vi "VI_Heat_Tape_Final_double.vi"() -> ()   [LabVIEW 2019]
uses:
  <vilib>/NI/Modbus Library/API/Wrapper/Create Serial Master.vi
  <vilib>/NI/Modbus Library/API/Master/Modbus Master.lvclass
  <vilib>/NI/Modbus Library/API/Wrapper/API Main.lvlib
  <vilib>/NI/Modbus Library/Transmission Data Unit/RTU/RTU Data Unit.lvclass
panel:
  in  "?":bool
  in  "unit ID (Defaut: 1) 2":u8=1
  in  "error check 2":errorcluster
  in  "Flow Control (Default: None) 2":u16(ring) items=["None", "XON/XOFF", "RTS/CTS", "XON/XOFF & RTS/CTS", "DTR/DSR", "XON/XOFF & DTR/DSR"]
  in  "Serial Type (Default: RTU) 2":enum16{"RTU", "ASCII"}(ring)
  in  "Parity (Default: None) 2":u16(ring)=2 items=["None", "Odd", "Even", "Mark", "Space"]
  in  "Baud Rate (Default: 115400) 2":u32=9600
  in  "COM Port (Default: COM7) 2":refnum<visa-resource-name>
  in  "starting address (Default: 1) 2":u16
  in  "number of inputs (Defaut: 60) 2":u16
  out "Register and RAW value 2":u16[](array[numeric])
  out "Query Message 2":string
  out "Heat Tape 01  Temperature (ºF) 2":dbl(slide) scale=65.0..85.0
  in  "?":bool
  out "Current Temperature (ºF) 2":string
  out "?":cluster{dbl, dbl}(graph)
  in  "Hysterisis Value 2":string
  out "Current Temperature Status 2":bool
  out "Alarm Status 2":bool
  out "Connection Status 2":bool
  in  "Manual/Auto 2":string(combo)
  in  "Set Value 2":string
  in  "Key Lock 2":string(combo)
  in  "Preset 2":string(combo)
  out "Heater Status 2":bool
  in  "Auto Tunning 2":string(combo)
  in  "Control Mode 2":string(combo)
  in  "?":bool
  in  "Normal/Reverse Setting 2":string(combo)
  in  "?":bool
  out "Value 5":sgl
  out "Value 4":sgl
  out "Value 3":sgl
  out "Value 2":sgl
  in  "Normal/Reverse Setting":string(combo)
  in  "Control Mode":string(combo)
  in  "Auto Tunning":string(combo)
  in  "?":bool
  in  "?":bool
  in  "Manual/Auto":string(combo)
  in  "Key Lock":string(combo)
  in  "Set Value":string
  in  "Preset":string(combo)
  in  "Hysterisis Value":string
  out "Connection Status":bool
  in  "unit ID (Defaut: 1)":u8=1
  in  "number of inputs (Defaut: 60)":u16
  in  "starting address (Default: 1)":u16
  in  "Flow Control (Default: None)":u16(ring) items=["None", "XON/XOFF", "RTS/CTS", "XON/XOFF & RTS/CTS", "DTR/DSR", "XON/XOFF & DTR/DSR"]
  in  "Serial Type (Default: RTU)":enum16{"RTU", "ASCII"}(ring)
  in  "Parity (Default: None)":u16(ring)=2 items=["None", "Odd", "Even", "Mark", "Space"]
  in  "Baud Rate (Default: 115400)":u32=9600
  in  "COM Port (Default: COM7)":refnum<visa-resource-name>
  out "Alarm Status":bool
  out "?":cluster{dbl, dbl}(graph)
  out "Heater Status":bool
  out "Current Temperature Status":bool
  in  "?":bool
  out "Current Temperature (ºF)":string
  out "Heat Tape 01  Temperature (ºF)":dbl(slide) scale=65.0..85.0
  out "Query Message":string
  out "Register and RAW value":u16[](array[numeric])
  in  "error check":errorcluster
  # "SpinQuest Heat Tape Temperature Monitoring System"
  # "PXF4 Settings"
  # "RS-485 Connection"
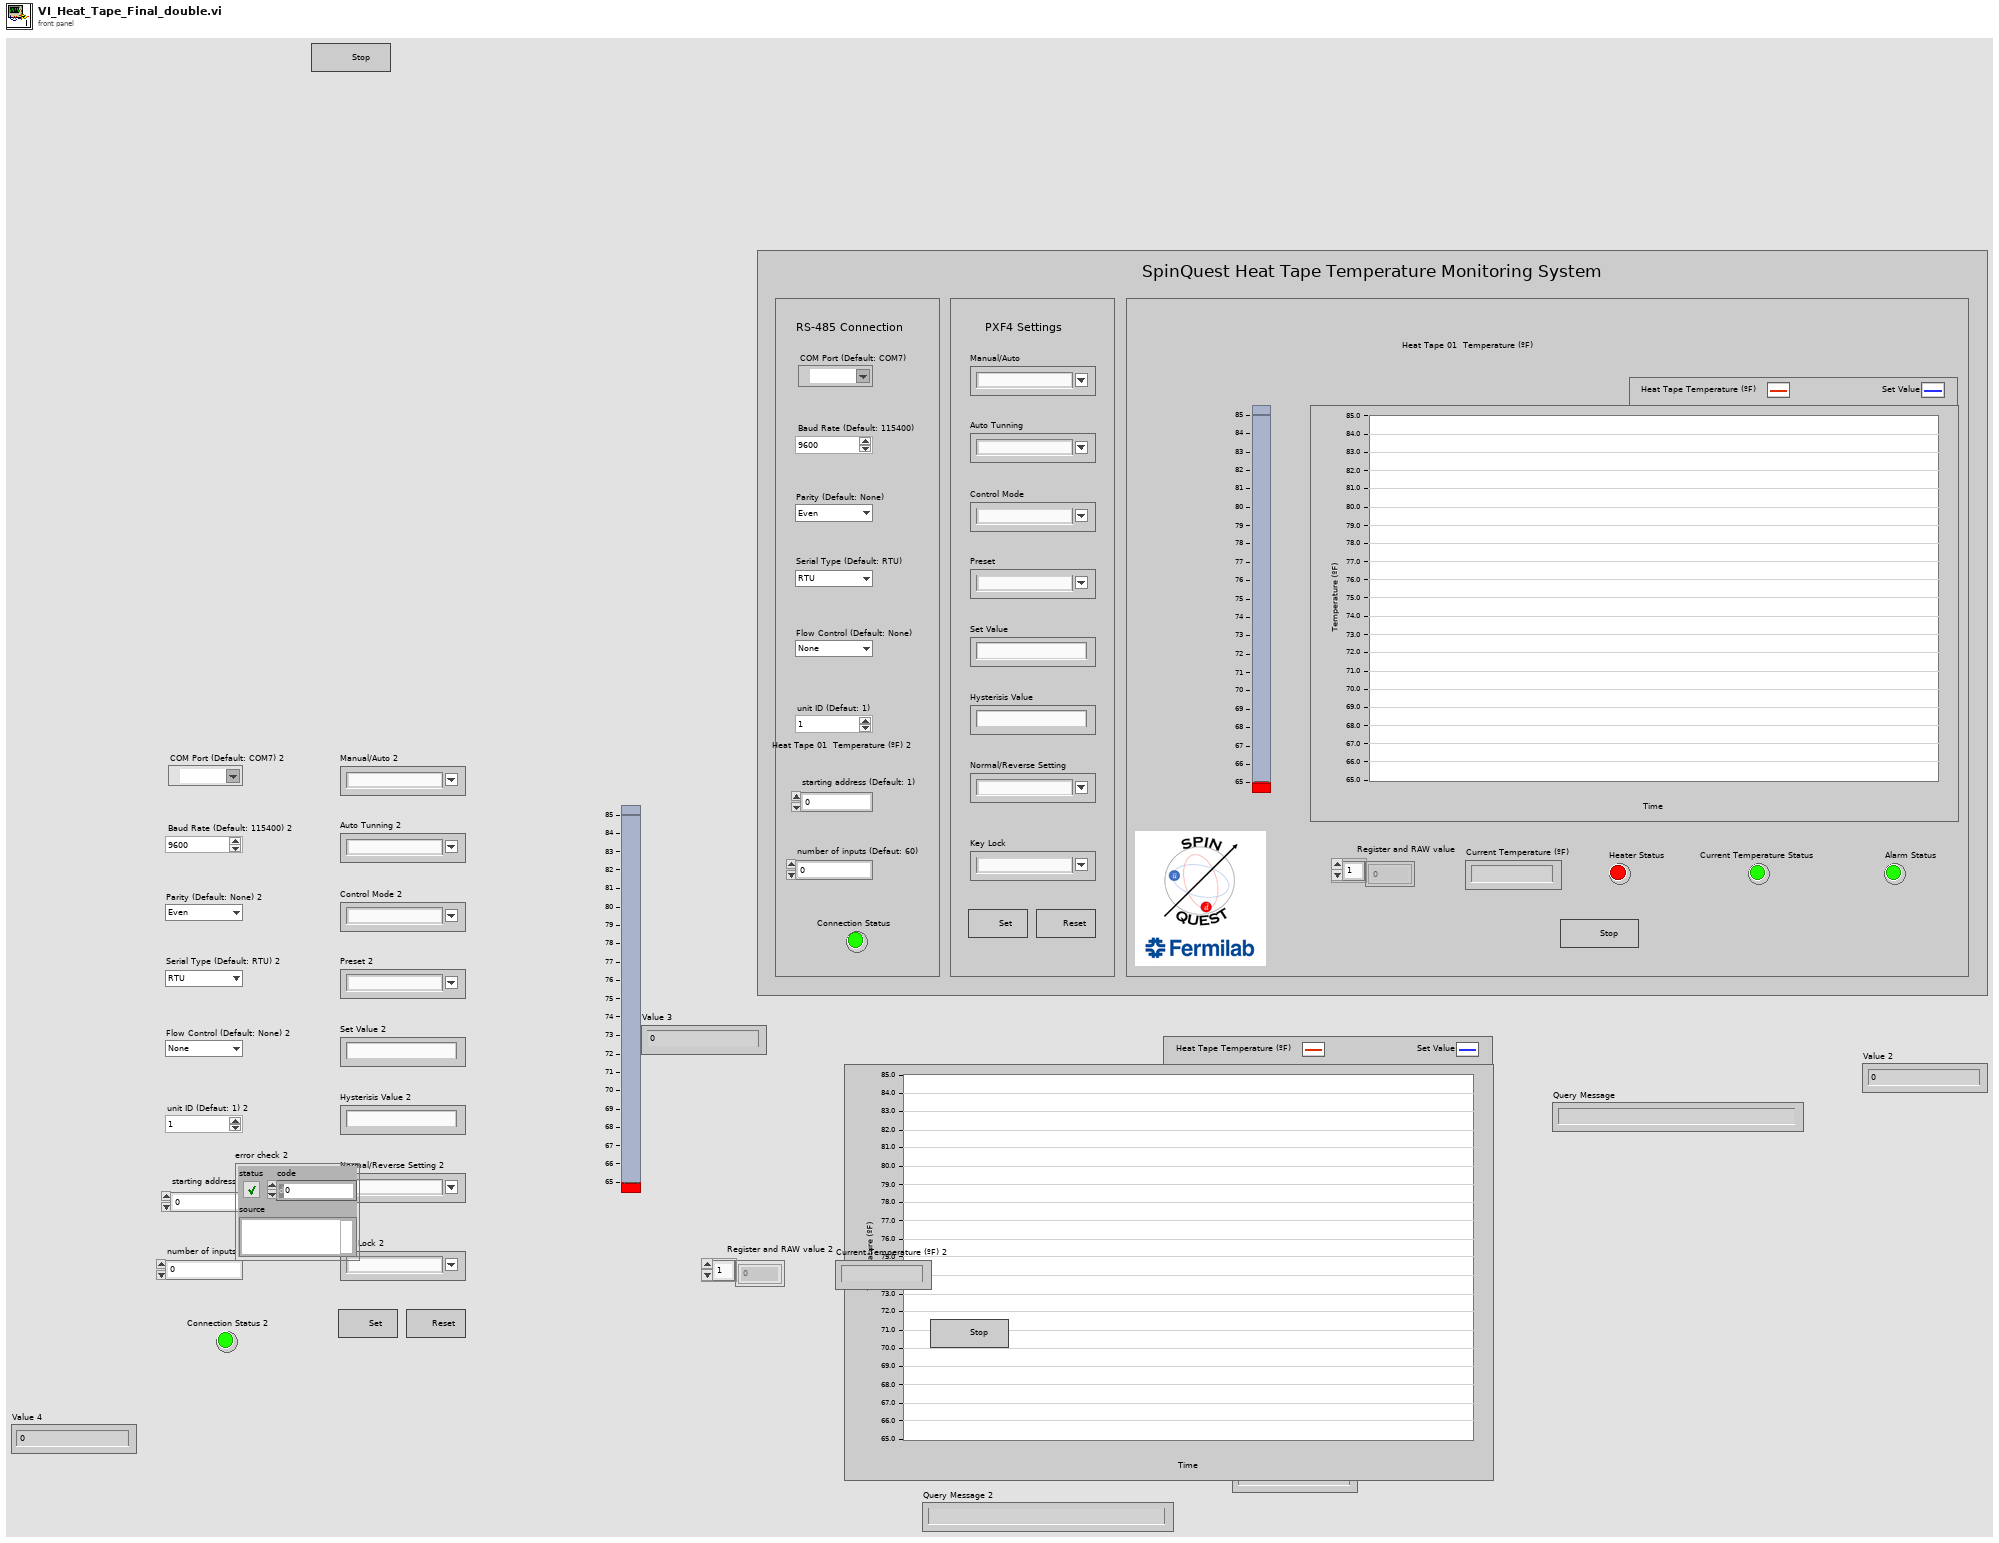
[diagram p1: front panel]
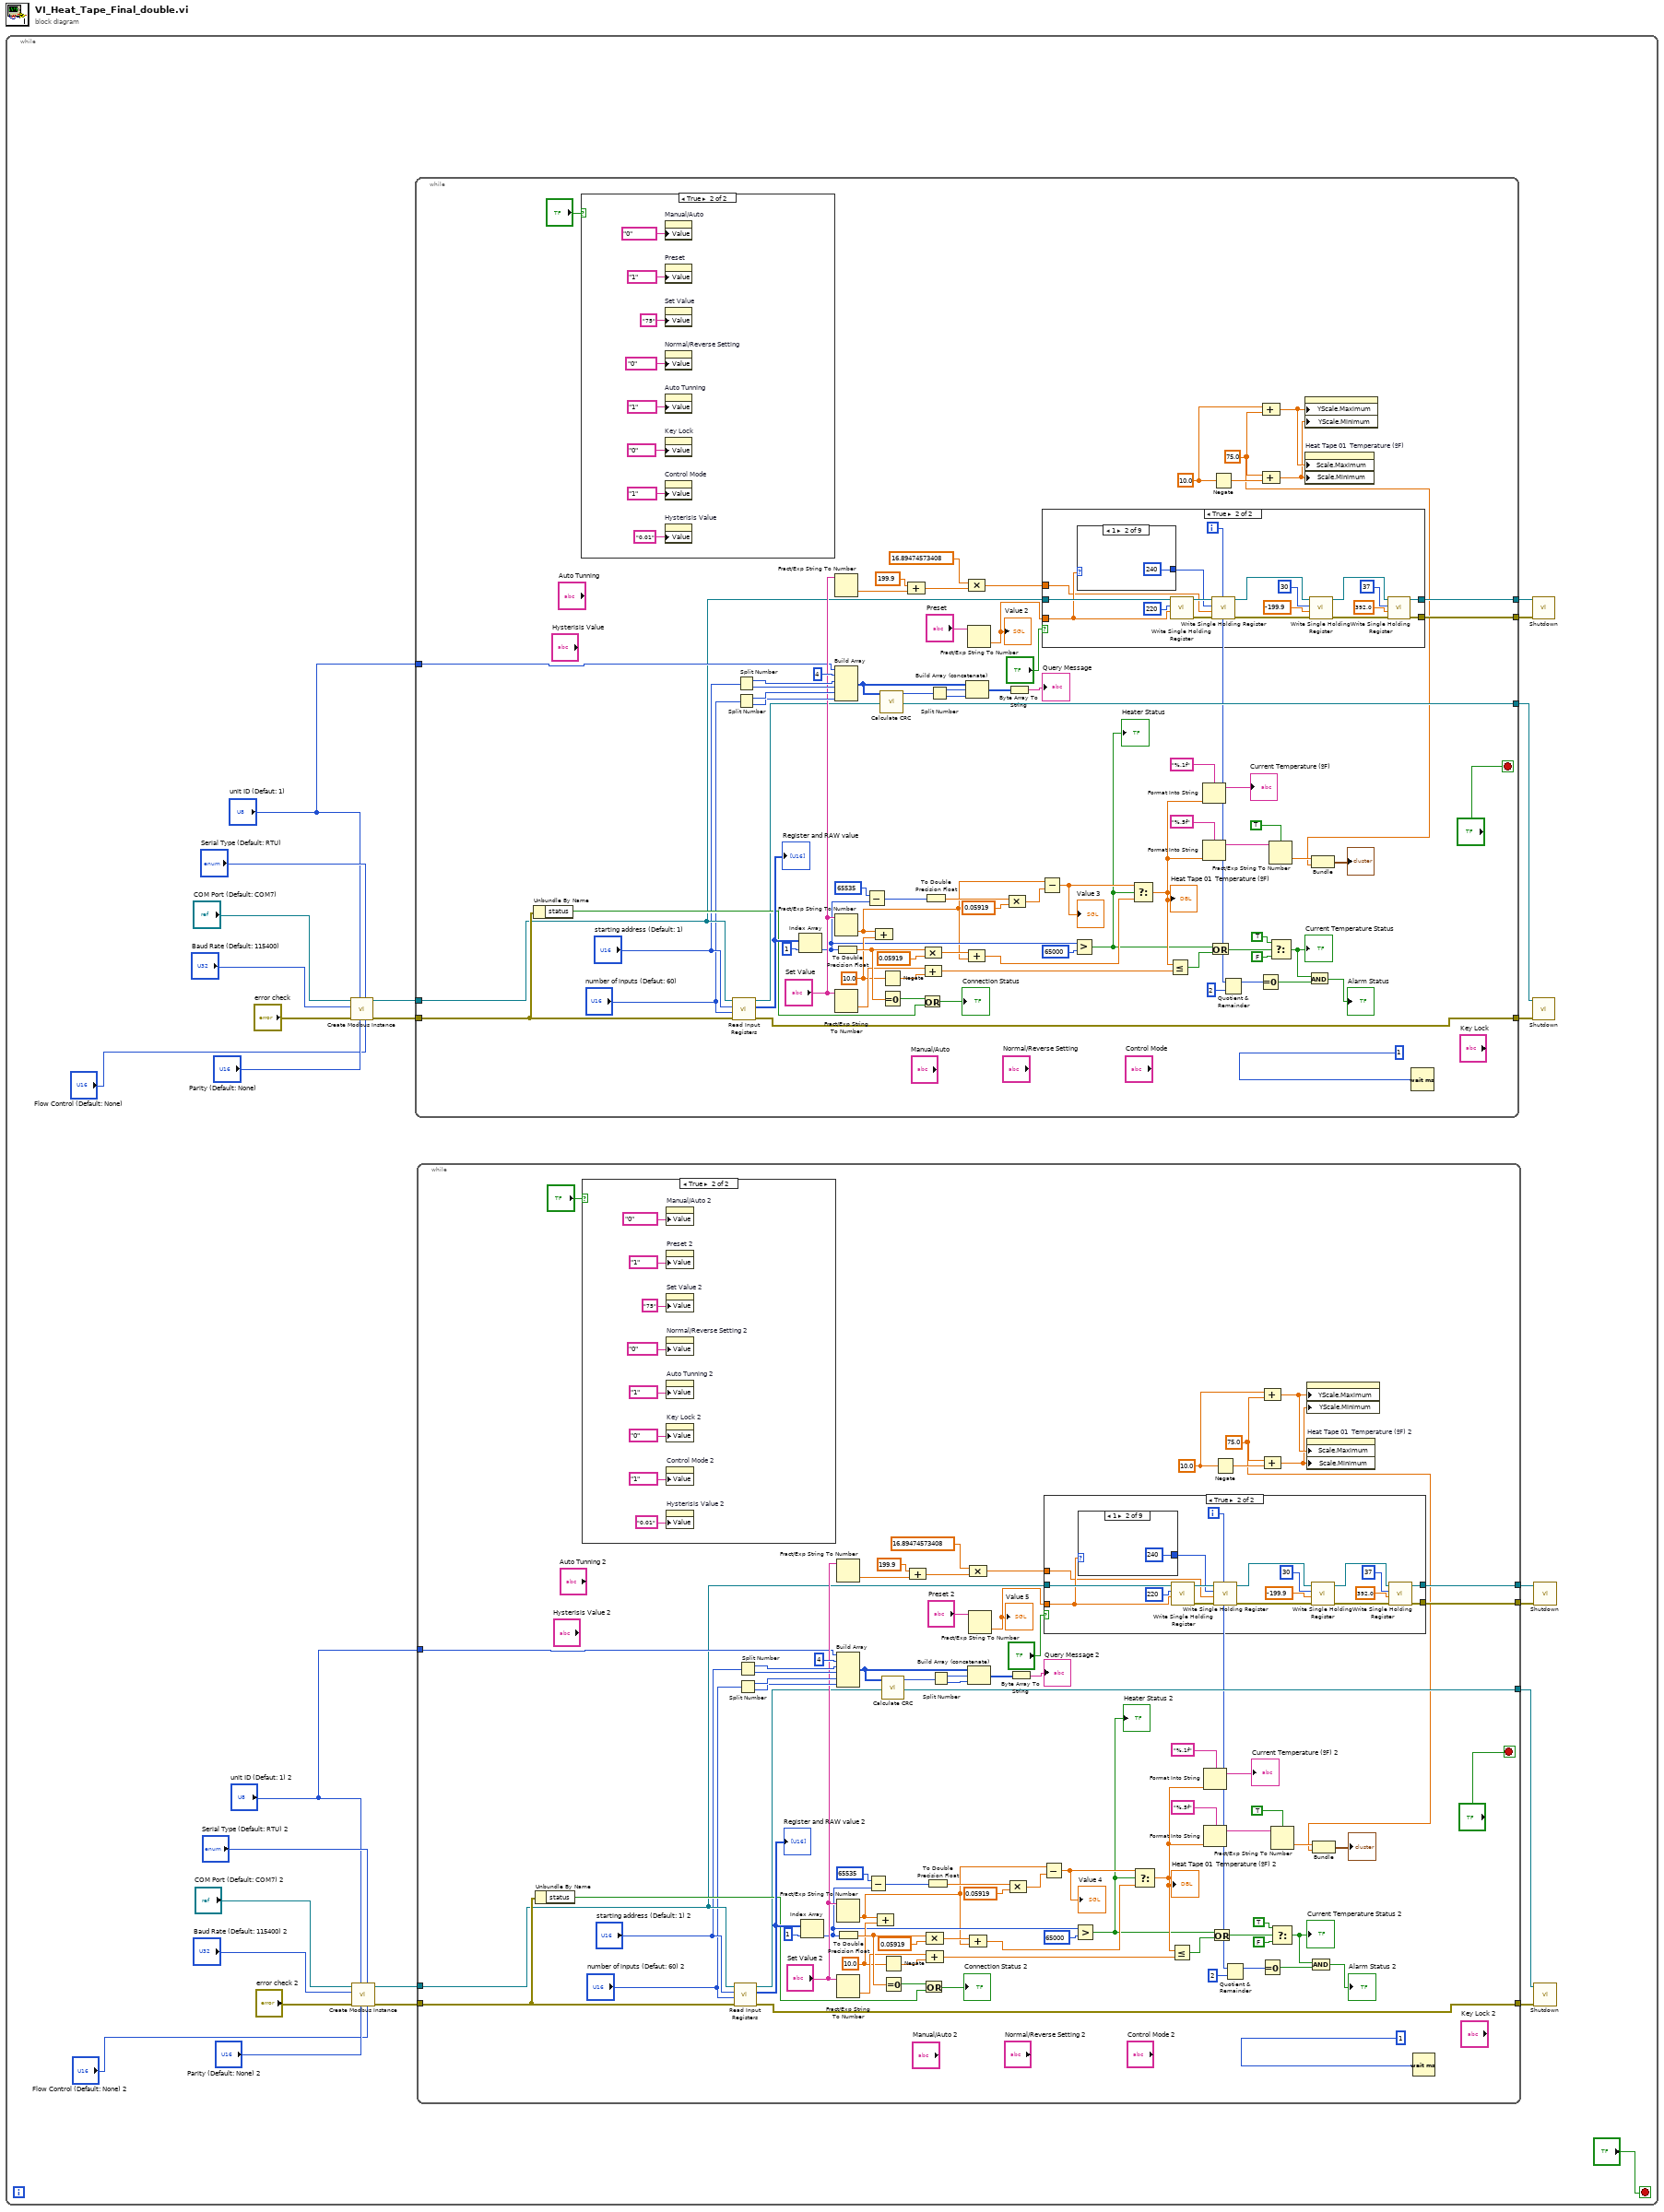
[diagram p0: block diagram]
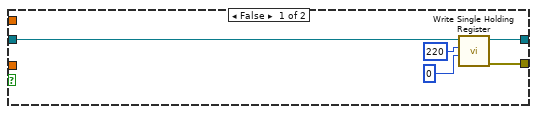
[diagram p2: hidden frame]
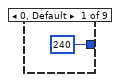
[diagram p3: hidden frame]
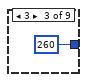
[diagram p4: hidden frame]
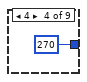
[diagram p5: hidden frame]
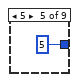
[diagram p6: hidden frame]
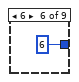
[diagram p7: hidden frame]
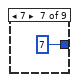
[diagram p8: hidden frame]
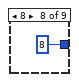
[diagram p9: hidden frame]
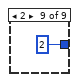
[diagram p10: hidden frame]
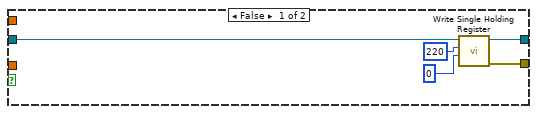
[diagram p12: hidden frame]
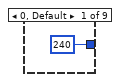
[diagram p13: hidden frame]
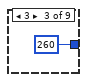
[diagram p14: hidden frame]
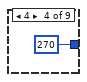
[diagram p15: hidden frame]
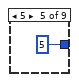
[diagram p16: hidden frame]
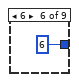
[diagram p17: hidden frame]
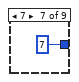
[diagram p18: hidden frame]
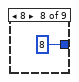
[diagram p19: hidden frame]
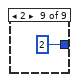
[diagram p20: hidden frame]
diagram:
  n1 = while {
    stop <- "?" stop-if-true
    n2 = call-poly <vilib>:"Create Modbus Instance.vi"("flow control (none)"="Flow Control (Default: None)", "serial type"="Serial Type (Default: RTU)", "parity (even)"="Parity (Default: None)", "unit ID"="unit ID (Defaut: 1)", "error in"="error check", "baud rate"="Baud Rate (Default: 115400)", "VISA resource name"="COM Port (Default: COM7)") -> ("error out"=w21:errorcluster, "serial master instance"=w22:refnum<class "Modbus Master.lvclass">)  [unwired: 3 in]
    n3 = call-poly <vilib>:"Create Modbus Instance.vi"("flow control (none)"="Flow Control (Default: None) 2", "serial type"="Serial Type (Default: RTU) 2", "parity (even)"="Parity (Default: None) 2", "unit ID"="unit ID (Defaut: 1) 2", "error in"="error check 2", "baud rate"="Baud Rate (Default: 115400) 2", "VISA resource name"="COM Port (Default: COM7) 2") -> ("error out"=w8:errorcluster, "serial master instance"=w9:refnum<class "Modbus Master.lvclass">)  [unwired: 3 in]
    n4 = while {
      tunnel: w22 -> [w147]
      tunnel: w21 -> [w191]
      tunnel: [w150] -> w19
      tunnel: [w151] -> w18
      tunnel: "unit ID (Defaut: 1)" -> [w152]
      tunnel: [w178] -> w17
      tunnel: [w177] -> w16
      i -> [w148]
      stop <- "?" stop-if-true
      w166 = 10.0 ("value")
      w149 = 75.0 ("value")
      w181 = 10.0 ("value")
      n5 = Unbundle By Name(w191) -> ("status"=w188:bool)
      n6 = case shown="True" "?" {
        frame False {
        }
        frame True {
          n7 = property on="Manual/Auto" class="CmbBox"("Value"="0" ("Manual/Auto")) -> ()  [unwired: 2 in, 2 out]
          n8 = property on="Preset" class="CmbBox"("Value"="1" ("Preset")) -> ()  [unwired: 2 in, 2 out]
          n9 = property on="Set Value" class="Str"("Value"="75" ("Set Value")) -> ()  [unwired: 2 in, 2 out]
          n10 = property on="Normal/Reverse Setting" class="CmbBox"("Value"="0" ("Normal/Reverse Setting")) -> ()  [unwired: 2 in, 2 out]
          n11 = property on="Auto Tunning" class="CmbBox"("Value"="1" ("Auto Tunning")) -> ()  [unwired: 2 in, 2 out]
          n12 = property on="Key Lock" class="CmbBox"("Value"="0" ("Key Lock")) -> ()  [unwired: 2 in, 2 out]
          n13 = property on="Control Mode" class="CmbBox"("Value"="1" ("Control Mode")) -> ()  [unwired: 2 in, 2 out]
          n14 = property on="Hysterisis Value" class="Str"("Value"="0.01" ("Hysterisis Value")) -> ()  [unwired: 2 in, 2 out]
        }
      }
      n15 = call-dynamic "Read Input Registers.vi"("error in"=w191, "number of inputs"="number of inputs (Defaut: 60)", "starting address"="starting address (Default: 1)", "Modbus master in"=w147) -> ("error out"=w150:errorcluster, "register values"=w209:u16[], "Modbus master out"=w151:refnum<class "Modbus Master.lvclass">)  [unwired: 5 in]
      "Register and RAW value" <- w209
      n16 = Split Number(x="starting address (Default: 1)") -> (hi(x)=w215:u8, lo(x)=w214:u8)
      n17 = Split Number(x="number of inputs (Defaut: 60)") -> (hi(x)=w213:u8, lo(x)=w212:u8)
      n18 = Index Array(array=w209, index=1) -> (element=w167:u16)
      n19 = Fract/Exp String To Number(string="Set Value") -> (number=w174:dbl)  [unwired: 3 in, 1 out]
      n20 = Build Array(w152, u8 4 ("element"), w215, w214, w213, w212) -> (w221:u8[])
      n21 = Fract/Exp String To Number(string="Set Value") -> (number=w156:dbl)  [unwired: 3 in, 1 out]
      n22 = Fract/Exp String To Number(string="Set Value") -> (number=w183:dbl)  [unwired: 3 in, 1 out]
      n23 = To Double Precision Float(number=w167) -> (double precision float=w190:dbl)
      n24 = Subtract(x=u16 65535 ("y"), y=w167) -> (x-y=w158:u16)
      n25 = Compound Arithmetic op=ADD(w156, w181) -> ()  [unwired: 1 out]
      n26 = call <vilib>:"Calculate CRC.vi"("data"=w221) -> ("CRC-16"=w220:u16)  [unwired: 10 in]
      n27 = Negate(x=w181) -> (-x=w180:dbl)
      n28 = Equal To 0?(x=w190) -> (x = 0?=w187:bool)
      n29 = Compound Arithmetic op=ADD(199.9 ("value"), w174) -> (w172:dbl)
      n30 = Or(x=w187, y=w188) -> (x .or. y?=→"Connection Status":bool)
      n31 = To Double Precision Float(number=w158) -> (double precision float=w160:dbl)
      n32 = Compound Arithmetic op=MULTIPLY(w190, 0.05919 ("value")) -> (w207:dbl)
      n33 = Compound Arithmetic op=ADD(w183, w180) -> (w162:dbl)
      n34 = Split Number(x=w220) -> (hi(x)=w219:u8, lo(x)=w218:u8)
      n35 = Build Array (concatenate)(w221, w219, w218) -> (w217:u8[])
      n36 = Fract/Exp String To Number(string="Preset") -> (number=w176:dbl)  [unwired: 3 in, 1 out]
      "Value 2" <- w176
      n37 = Compound Arithmetic op=MULTIPLY(16.89474573408 ("value"), w172) -> (w170:dbl)
      n38 = Compound Arithmetic op=ADD(w207, w156) -> (w154:dbl)
      n39 = Byte Array To String(unsigned byte array=w217) -> (string=→"Query Message":string)
      n40 = Compound Arithmetic op=MULTIPLY(w160, 0.05919 ("value")) -> (w157:dbl)
      n41 = Subtract(x=w156, y=w157) -> (x-y=w155:dbl)
      "Value 3" <- w155
      n42 = case shown="True" "?" {
        tunnel: w147 -> [w225 w244]
        tunnel: [w226 w232] -> w178
        tunnel: [w227 w231] -> w177
        tunnel: w176 -> [_ w242]
        tunnel: w170 -> [_ w239]
        frame False {
          n43 = call-dynamic "Write Single Holding Register.vi"("register to write"=u16 0, "address"=u16 220, "Modbus master in"=w225) -> ("error out"=w227:errorcluster, "Modbus master out"=w226:refnum<class "Modbus Master.lvclass">)  [unwired: 7 in]
        }
        frame True {
          n44 = case shown="1" w242 {
            tunnel: [240 240 260 270 5 6 7 8 2] -> w238
            frame 0, Default {
            }
            frame 1 {
            }
            frame 3 {
            }
            frame 4 {
            }
            frame 5 {
            }
            frame 6 {
            }
            frame 7 {
            }
            frame 8 {
            }
            frame 2 {
            }
          }
          n45 = call-dynamic "Write Single Holding Register.vi"("register to write"=w242, "address"=u16 220, "Modbus master in"=w244) -> ("error out"=w240:errorcluster, "Modbus master out"=w241:refnum<class "Modbus Master.lvclass">)  [unwired: 7 in]
          n46 = call-dynamic "Write Single Holding Register.vi"("error in"=w240, "register to write"=w239, "address"=w238, "Modbus master in"=w241) -> ("error out"=w236:errorcluster, "Modbus master out"=w237:refnum<class "Modbus Master.lvclass">)  [unwired: 6 in]
          n47 = call-dynamic "Write Single Holding Register.vi"("error in"=w236, "register to write"=-199.9 ("value"), "address"=u16 30, "Modbus master in"=w237) -> ("error out"=w234:errorcluster, "Modbus master out"=w233:refnum<class "Modbus Master.lvclass">)  [unwired: 6 in]
          n48 = call-dynamic "Write Single Holding Register.vi"("error in"=w234, "register to write"=392.0 ("value"), "address"=u16 37, "Modbus master in"=w233) -> ("error out"=w231:errorcluster, "Modbus master out"=w232:refnum<class "Modbus Master.lvclass">)  [unwired: 6 in]
        }
      }
      n49 = Greater?(x=w167, y=u16 65000) -> (0:w153:bool)
      "Heater Status" <- w153
      n50 = Select(t=w155, s=w153, f=w154) -> (s? t:f=w161:dbl)
      "Heat Tape 01  Temperature (ºF)" <- w161
      n51 = Less Or Equal?(x=w161, y=w162) -> (x <= y?=w200:bool)
      n52 = Format Into String(format string="%.1f", w161) -> (resulting string=→"Current Temperature (ºF)":string)  [unwired: 2 in, 1 out]
      n53 = Format Into String(format string="%.5f", w161) -> (resulting string=w202:string)  [unwired: 2 in, 1 out]
      n54 = Or(x=w153, y=w200) -> (x .or. y?=w199:bool)
      n55 = Negate(x=w166) -> (-x=w165:dbl)
      n56 = Quotient & Remainder(x=w148, y=2) -> (x-y*floor(x/y)=w196:i32)  [unwired: 1 out]
      n57 = Equal To 0?(x=w196) -> (x = 0?=w194:bool)
      n58 = Compound Arithmetic op=unknown(w166, w149) -> (w164:dbl)
      n59 = Compound Arithmetic op=unknown(w149, w165) -> (w163:dbl)
      n60 = Fract/Exp String To Number(use system decimal point (T)=TRUE, string=w202) -> (number=w185:dbl)  [unwired: 2 in, 1 out]
      n61 = Select(t=TRUE, s=w199, f=FALSE) -> (s? t:f=w193:bool)
      "Current Temperature Status" <- w193
      n62 = property class="WFChart (strict)"("YScale.Maximum"=w164, "YScale.Minimum"=w163) -> ()  [unwired: 2 in, 2 out]
      n63 = property on="Heat Tape 01  Temperature (ºF)" class="Slide (strict)"("Scale.Maximum"=w164, "Scale.Minimum"=w163) -> ()  [unwired: 2 in, 2 out]
      n64 = And(x=w193, y=w194) -> (x .and. y?=→"Alarm Status":bool)
      n65 = Bundle(w185, "value"=w149) -> (→"?":cluster{dbl, "value":dbl})  [unwired: 1 in]
      n66 = Wait (ms)(milliseconds to wait=u32 1) -> ()  [unwired: 1 out]
    }
    n67 = while {
      tunnel: w9 -> [w30]
      tunnel: w8 -> [w74]
      tunnel: [w33] -> w6
      tunnel: [w34] -> w5
      tunnel: "unit ID (Defaut: 1) 2" -> [w35]
      tunnel: [w61] -> w4
      tunnel: [w60] -> w3
      i -> [w31]
      stop <- "?" stop-if-true
      w49 = 10.0 ("value")
      w32 = 75.0 ("value")
      w64 = 10.0 ("value")
      n68 = Unbundle By Name(w74) -> ("status"=w71:bool)
      n69 = case shown="True" "?" {
        frame False {
        }
        frame True {
          n70 = property on="Manual/Auto 2" class="CmbBox"("Value"="0" ("Manual/Auto")) -> ()  [unwired: 2 in, 2 out]
          n71 = property on="Preset 2" class="CmbBox"("Value"="1" ("Preset")) -> ()  [unwired: 2 in, 2 out]
          n72 = property on="Set Value 2" class="Str"("Value"="75" ("Set Value")) -> ()  [unwired: 2 in, 2 out]
          n73 = property on="Normal/Reverse Setting 2" class="CmbBox"("Value"="0" ("Normal/Reverse Setting")) -> ()  [unwired: 2 in, 2 out]
          n74 = property on="Auto Tunning 2" class="CmbBox"("Value"="1" ("Auto Tunning")) -> ()  [unwired: 2 in, 2 out]
          n75 = property on="Key Lock 2" class="CmbBox"("Value"="0" ("Key Lock")) -> ()  [unwired: 2 in, 2 out]
          n76 = property on="Control Mode 2" class="CmbBox"("Value"="1" ("Control Mode")) -> ()  [unwired: 2 in, 2 out]
          n77 = property on="Hysterisis Value 2" class="Str"("Value"="0.01" ("Hysterisis Value")) -> ()  [unwired: 2 in, 2 out]
        }
      }
      n78 = call-dynamic "Read Input Registers.vi"("error in"=w74, "number of inputs"="number of inputs (Defaut: 60) 2", "starting address"="starting address (Default: 1) 2", "Modbus master in"=w30) -> ("error out"=w33:errorcluster, "register values"=w92:u16[], "Modbus master out"=w34:refnum<class "Modbus Master.lvclass">)  [unwired: 5 in]
      "Register and RAW value 2" <- w92
      n79 = Split Number(x="starting address (Default: 1) 2") -> (hi(x)=w98:u8, lo(x)=w97:u8)
      n80 = Split Number(x="number of inputs (Defaut: 60) 2") -> (hi(x)=w96:u8, lo(x)=w95:u8)
      n81 = Index Array(array=w92, index=1) -> (element=w50:u16)
      n82 = Fract/Exp String To Number(string="Set Value 2") -> (number=w57:dbl)  [unwired: 3 in, 1 out]
      n83 = Build Array(w35, u8 4 ("element"), w98, w97, w96, w95) -> (w104:u8[])
      n84 = Fract/Exp String To Number(string="Set Value 2") -> (number=w39:dbl)  [unwired: 3 in, 1 out]
      n85 = Fract/Exp String To Number(string="Set Value 2") -> (number=w66:dbl)  [unwired: 3 in, 1 out]
      n86 = To Double Precision Float(number=w50) -> (double precision float=w73:dbl)
      n87 = Subtract(x=u16 65535 ("y"), y=w50) -> (x-y=w41:u16)
      n88 = Compound Arithmetic op=ADD(w39, w64) -> ()  [unwired: 1 out]
      n89 = call <vilib>:"Calculate CRC.vi"("data"=w104) -> ("CRC-16"=w103:u16)  [unwired: 10 in]
      n90 = Negate(x=w64) -> (-x=w63:dbl)
      n91 = Equal To 0?(x=w73) -> (x = 0?=w70:bool)
      n92 = Compound Arithmetic op=ADD(199.9 ("value"), w57) -> (w55:dbl)
      n93 = Or(x=w70, y=w71) -> (x .or. y?=→"Connection Status 2":bool)
      n94 = To Double Precision Float(number=w41) -> (double precision float=w43:dbl)
      n95 = Compound Arithmetic op=MULTIPLY(w73, 0.05919 ("value")) -> (w90:dbl)
      n96 = Compound Arithmetic op=ADD(w66, w63) -> (w45:dbl)
      n97 = Split Number(x=w103) -> (hi(x)=w102:u8, lo(x)=w101:u8)
      n98 = Build Array (concatenate)(w104, w102, w101) -> (w100:u8[])
      n99 = Fract/Exp String To Number(string="Preset 2") -> (number=w59:dbl)  [unwired: 3 in, 1 out]
      "Value 5" <- w59
      n100 = Compound Arithmetic op=MULTIPLY(16.89474573408 ("value"), w55) -> (w53:dbl)
      n101 = Compound Arithmetic op=ADD(w90, w39) -> (w37:dbl)
      n102 = Byte Array To String(unsigned byte array=w100) -> (string=→"Query Message 2":string)
      n103 = Compound Arithmetic op=MULTIPLY(w43, 0.05919 ("value")) -> (w40:dbl)
      n104 = Subtract(x=w39, y=w40) -> (x-y=w38:dbl)
      "Value 4" <- w38
      n105 = case shown="True" "?" {
        tunnel: w30 -> [w108 w127]
        tunnel: [w109 w115] -> w61
        tunnel: [w110 w114] -> w60
        tunnel: w59 -> [_ w125]
        tunnel: w53 -> [_ w122]
        frame False {
          n106 = call-dynamic "Write Single Holding Register.vi"("register to write"=u16 0, "address"=u16 220, "Modbus master in"=w108) -> ("error out"=w110:errorcluster, "Modbus master out"=w109:refnum<class "Modbus Master.lvclass">)  [unwired: 7 in]
        }
        frame True {
          n107 = case shown="1" w125 {
            tunnel: [240 240 260 270 5 6 7 8 2] -> w121
            frame 0, Default {
            }
            frame 1 {
            }
            frame 3 {
            }
            frame 4 {
            }
            frame 5 {
            }
            frame 6 {
            }
            frame 7 {
            }
            frame 8 {
            }
            frame 2 {
            }
          }
          n108 = call-dynamic "Write Single Holding Register.vi"("register to write"=w125, "address"=u16 220, "Modbus master in"=w127) -> ("error out"=w123:errorcluster, "Modbus master out"=w124:refnum<class "Modbus Master.lvclass">)  [unwired: 7 in]
          n109 = call-dynamic "Write Single Holding Register.vi"("error in"=w123, "register to write"=w122, "address"=w121, "Modbus master in"=w124) -> ("error out"=w119:errorcluster, "Modbus master out"=w120:refnum<class "Modbus Master.lvclass">)  [unwired: 6 in]
          n110 = call-dynamic "Write Single Holding Register.vi"("error in"=w119, "register to write"=-199.9 ("value"), "address"=u16 30, "Modbus master in"=w120) -> ("error out"=w117:errorcluster, "Modbus master out"=w116:refnum<class "Modbus Master.lvclass">)  [unwired: 6 in]
          n111 = call-dynamic "Write Single Holding Register.vi"("error in"=w117, "register to write"=392.0 ("value"), "address"=u16 37, "Modbus master in"=w116) -> ("error out"=w114:errorcluster, "Modbus master out"=w115:refnum<class "Modbus Master.lvclass">)  [unwired: 6 in]
        }
      }
      n112 = Greater?(x=w50, y=u16 65000) -> (0:w36:bool)
      "Heater Status 2" <- w36
      n113 = Select(t=w38, s=w36, f=w37) -> (s? t:f=w44:dbl)
      "Heat Tape 01  Temperature (ºF) 2" <- w44
      n114 = Less Or Equal?(x=w44, y=w45) -> (x <= y?=w83:bool)
      n115 = Format Into String(format string="%.1f", w44) -> (resulting string=→"Current Temperature (ºF) 2":string)  [unwired: 2 in, 1 out]
      n116 = Format Into String(format string="%.5f", w44) -> (resulting string=w85:string)  [unwired: 2 in, 1 out]
      n117 = Or(x=w36, y=w83) -> (x .or. y?=w82:bool)
      n118 = Negate(x=w49) -> (-x=w48:dbl)
      n119 = Quotient & Remainder(x=w31, y=2) -> (x-y*floor(x/y)=w79:i32)  [unwired: 1 out]
      n120 = Equal To 0?(x=w79) -> (x = 0?=w77:bool)
      n121 = Compound Arithmetic op=unknown(w49, w32) -> (w47:dbl)
      n122 = Compound Arithmetic op=unknown(w32, w48) -> (w46:dbl)
      n123 = Fract/Exp String To Number(use system decimal point (T)=TRUE, string=w85) -> (number=w68:dbl)  [unwired: 2 in, 1 out]
      n124 = Select(t=TRUE, s=w82, f=FALSE) -> (s? t:f=w76:bool)
      "Current Temperature Status 2" <- w76
      n125 = property class="WFChart (strict)"("YScale.Maximum"=w47, "YScale.Minimum"=w46) -> ()  [unwired: 2 in, 2 out]
      n126 = property on="Heat Tape 01  Temperature (ºF) 2" class="Slide (strict)"("Scale.Maximum"=w47, "Scale.Minimum"=w46) -> ()  [unwired: 2 in, 2 out]
      n127 = And(x=w76, y=w77) -> (x .and. y?=→"Alarm Status 2":bool)
      n128 = Bundle(w68, "value"=w32) -> (→"?":cluster{dbl, "value":dbl})  [unwired: 1 in]
      n129 = Wait (ms)(milliseconds to wait=u32 1) -> ()  [unwired: 1 out]
    }
    n130 = call-dynamic "Shutdown.vi"("error in"=w16, "Modbus master in"=w17) -> ()  [unwired: 9 in, 1 out]
    n131 = call-dynamic "Shutdown.vi"("error in"=w19, "Modbus master in"=w18) -> ()  [unwired: 9 in, 1 out]
    n132 = call-dynamic "Shutdown.vi"("error in"=w3, "Modbus master in"=w4) -> ()  [unwired: 9 in, 1 out]
    n133 = call-dynamic "Shutdown.vi"("error in"=w6, "Modbus master in"=w5) -> ()  [unwired: 9 in, 1 out]
  }
